vi "Robot Main.vi"   [LabVIEW 2011]
doc: "This VI imlements the framework and scheduler for your robotics program. It should not be necessary to modify the framework. You are expected to add your code to the VIs called from Robot Main, the ones located in the Team Code within the project."
panel:
  # "THUNDER"
  # "you've been...THUNDERSTRUCK!"
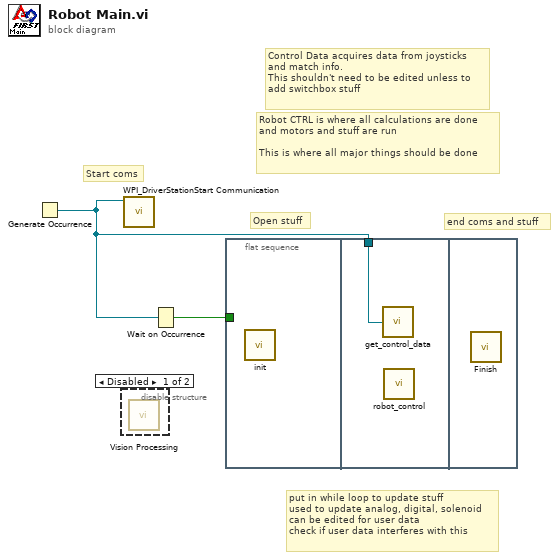
[diagram p0: block diagram]
diagram:
  # "put in while loop to update stuff\nused to update analog, digital, solenoid\ncan be edited for user data\ncheck if user data interferes with this"
  # "Robot CTRL is where all calculations are done\nand motors and stuff are run\n\nThis is where all major things should be done"
  # "Control Data acquires data from joysticks\nand match info.\nThis shouldn't need to be edited unless to\nadd switchbox stuff"
  # "Open stuff"
  # "end coms and stuff"
  # "Start coms"
  n1 = Generate Occurrence() -> (w1:refnum<k4>)
  n2 = disable-structure shown="Disabled" {
    frame Disabled {
      n3 = call "Vision Processing.vi"() -> ()  [unwired: 1 in, 7 out]
    }
    frame Enabled {
    }
  }
  n4 = call <vilib>:"WPI_DriverStationStart Communication.vi"("occurrence"=w1) -> ()  [unwired: 11 out]
  n5 = Wait on Occurrence(2:w1) -> (0:w2:bool)  [unwired: 2 out]
  n6 = flat-sequence {
    tunnel: w2 -> [_]
    tunnel: w1 -> [w3]
    frame #0 {
      n7 = call "init.vi"() -> ()  [unwired: 12 out]
    }
    frame #1 {
      n8 = call "get_control_data.vi"("DS Occurrence"=w3) -> ()  [unwired: 1 in]
      n9 = call "robot_control.vi"() -> ()  [unwired: 1 out]
    }
    frame #2 {
      n10 = call "Finish.vi"() -> ()  [unwired: 8 out]
    }
  }
